vi "ReadCom2.vi"(8 "error in (no error)":errorcluster, 11 "Data In":T1) -> (0 "error out":errorcluster, 3 "Data Out":T1)   [LabVIEW 2014]
uses:
  controls/Data.ctl
  controls/ReadScan1States.ctl
panel:
  # "日期"
  # "機種名稱"
  # "機種代號"
  # "商品條碼"
  # "台"
  # "OK"
  # "NG"
  # "台"
  # "總計"
  # "台"
  # "日期"
  # "機種名稱"
  # "機種代號"
  # "商品條碼"
  # "台"
  # "OK"
  # "NG"
  # "台"
  # "總計"
  # "台"
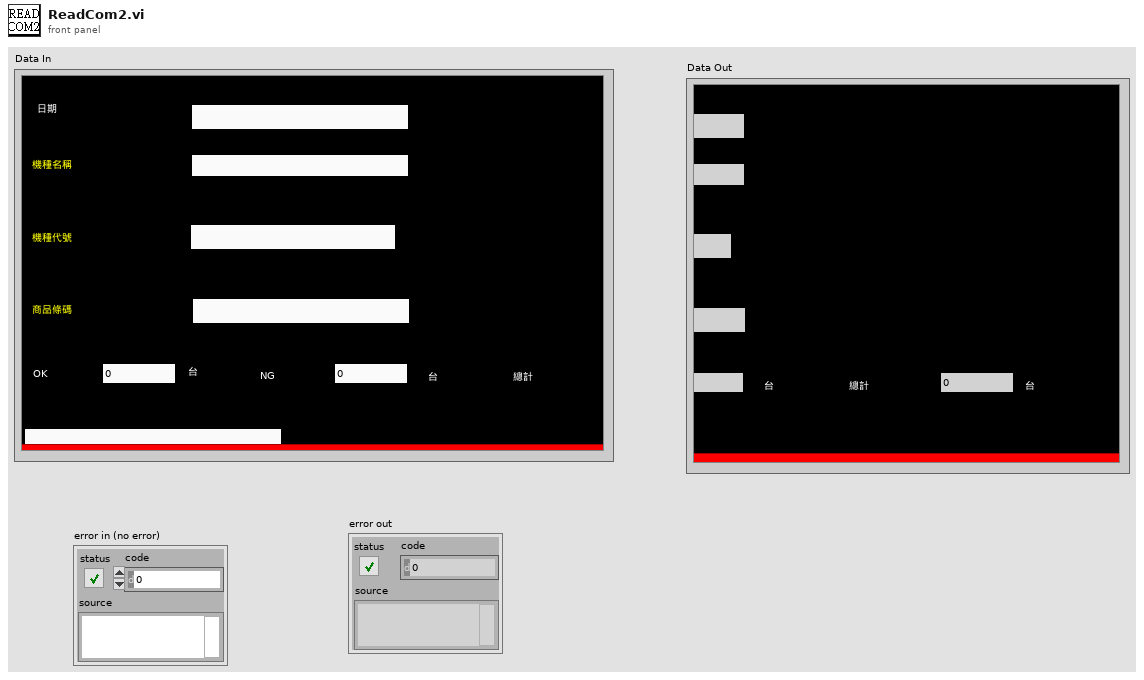
[diagram p1: front panel]
types:
  T1 = typedef "Data.ctl" = cluster{"Date":string, "BarCode1":string, "BarCode2":string, "BarCode3":string, "Message":string, "OK Count":u16, "NG Count":u16, "Total Count":u16, "ModelData":string[][], "OK&NG":bool, "COM1":refnum<visa-resource-name>, "COM2":refnum<visa-resource-name>, "IO":i32, "Time":u32, "TCP":refnum<k5>, "TCP 2":refnum<k5>, "COM3":refnum<visa-resource-name>}
  T2 = typedef "ReadScan1States.ctl" = enum16{"Initialize", "Init2", "Step1", "Step2", "Step3", "Step4", "One", "Two", "Three", "Four", "Five", "End", "Stop"}
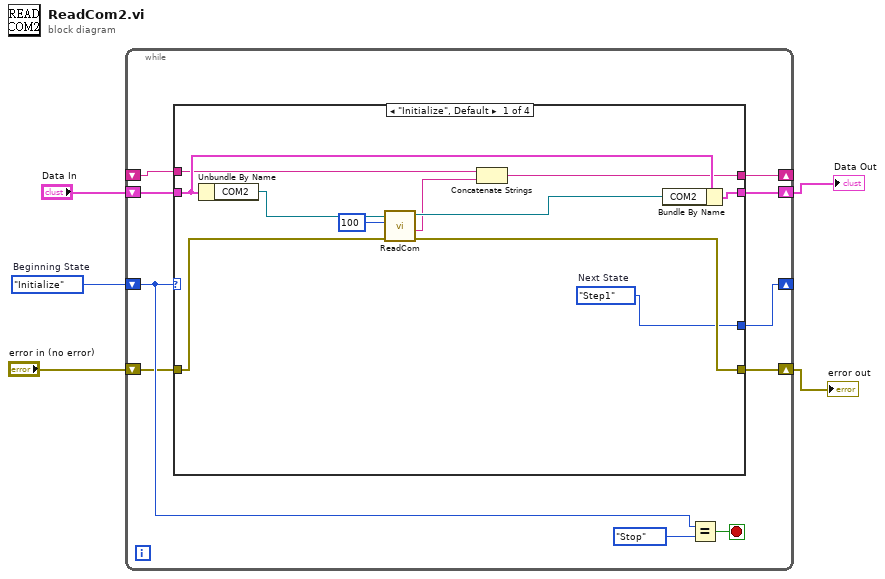
[diagram p0: block diagram]
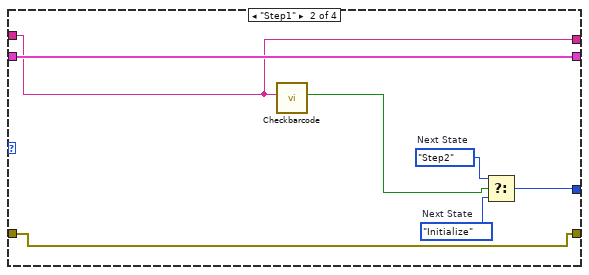
[diagram p2: hidden frame]
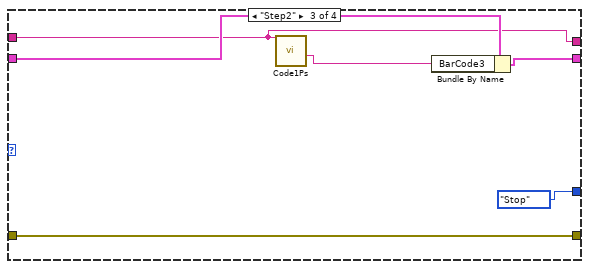
[diagram p3: hidden frame]
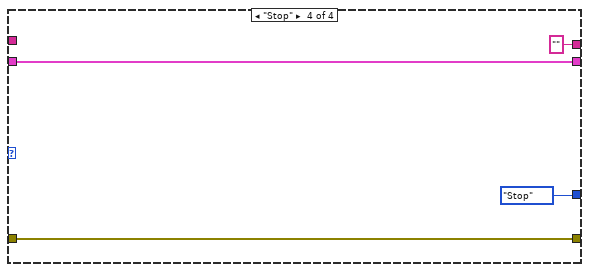
[diagram p4: hidden frame]
diagram:
  w5 = ReadScan1States."Initialize"  # Beginning State
  n1 = while {
    shift-right: [w12] -> _
    shift-left: w5 -> [w14]
    shift-right: [w10] -> w3
    shift-left: "Data In" -> [w11]
    shift-right: [w9] -> _
    shift-left: _ -> [w8]
    shift-right: [w6] -> w1
    shift-left: "error in (no error)" -> [w7]
    stop <- w13 stop-if-true
    n2 = case shown="\"Initialize\", Default" w14 {
      tunnel: [w16 w31 ReadScan1States."Stop" ("States") ReadScan1States."Stop" ("States")] -> w12
      tunnel: w11 -> [w26 w29 w38 w42]
      tunnel: [w25 w29 w37 w42] -> w10
      tunnel: [w17 w28 w36 ""] -> w9
      tunnel: w8 -> [w20 w28 w36 _]
      tunnel: w7 -> [w19 w27 w35 w40]
      tunnel: [w18 w27 w35 w40] -> w6
      frame "Initialize", Default {
        w16 = ReadScan1States."Step1"  # Next State
        n3 = Unbundle By Name(w26) -> ("COM2"=w23:refnum<visa-resource-name>)
        n4 = call "ReadCom.vi"("error in (no error)"=w19, "delay before read (ms)"=u32 100, "Com In"=w23) -> ("error out"=w18:errorcluster, "Response"=w21:string, "Com Out"=w22:refnum<visa-resource-name>)  [unwired: 5 in, 1 out]
        n5 = Concatenate Strings(w20, w21) -> (w17:string)
        n6 = Bundle By Name(cluster=w26, "COM2"=w22) -> (w25:T1)
      }
      frame "Step1" {
        w32 = ReadScan1States."Step2"  # Next State
        w33 = ReadScan1States."Initialize"  # Next State
        n7 = call "Checkbarcode.vi"("String In"=w28) -> ("Complete"=w30:bool)  [unwired: 10 in]
        n8 = Select(t=w32, s=w30, f=w33) -> (s? t:f=w31:T2)
      }
      frame "Step2" {
        n9 = call "Code1Ps.vi"("Code1 In"=w36) -> ("紙箱號碼"=w39:string)  [unwired: 8 in, 2 out]
        n10 = Bundle By Name(cluster=w38, "BarCode3"=w39) -> (w37:T1)
      }
      frame "Stop" {
      }
    }
    n11 = Equal?(x=w14, y=ReadScan1States."Stop" ("States")) -> (x = y?=w13:bool)
  }
  "Data Out" <- w3
  "error out" <- w1
